vi "Read Occupied Queue.vi"(8 "error in (no error)":errorcluster, 11 "Circular Buffer 2D U16 DVR Queue Circular Buffer in":refnum<class "Circular Buffer 2D U16 DVR Queue Circular Buffer.lvclass">) -> (0 "error out":errorcluster, 2 "2D U16 DVR Queue":T1, 3 "Circular Buffer 2D U16 DVR Queue Circular Buffer out":refnum<class "Circular Buffer 2D U16 DVR Queue Circular Buffer.lvclass">)   [LabVIEW 2024, in "Circular Buffer 2D U16 DVR Queue Circular Buffer.lvclass"]
uses:
  Circular Buffer 2D U16 DVR Queue Circular Buffer.lvclass
  Type Def/2D U16 DVR Queue.ctl
  Type Def/2D U16 DVR.ctl
  Circular Buffer 2D U16 DVR Queue Circular Buffer.lvclass/Circular Buffer 2D U16 DVR Queue Circular Buffer.ctl
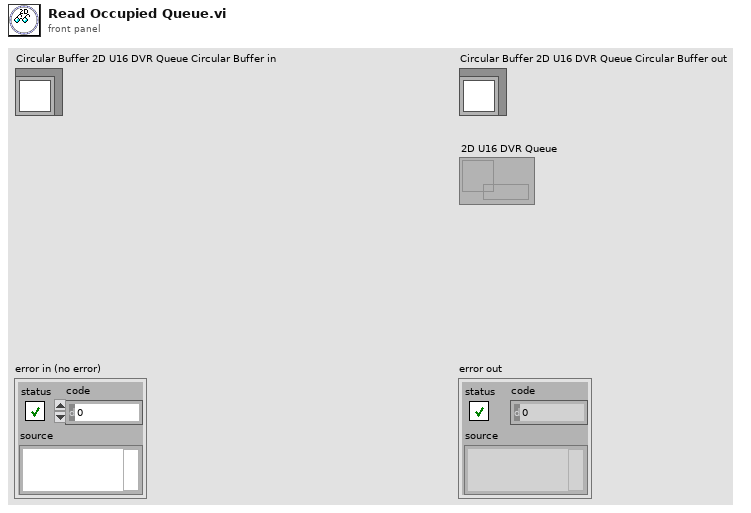
[diagram p1: front panel]
types:
  T1 = typedef "2D U16 DVR Queue.ctl" = refnum<queue>
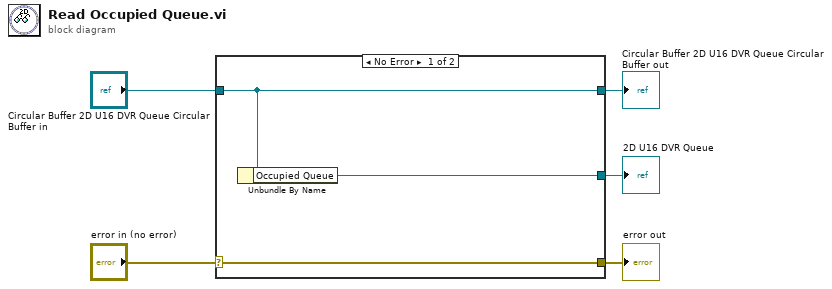
[diagram p0: block diagram]
diagram:
  n1 = case shown="No Error" "error in (no error)" {
    selector: "error in (no error)" -> [w8 w9]
    tunnel: [w8 w9] -> w4
    tunnel: [w7 w10] -> w2
    tunnel: "Circular Buffer 2D U16 DVR Queue Circular Buffer in" -> [w7 w10]
    tunnel: [w6 _] -> w1
    frame No Error {
      n2 = Unbundle By Name(w7) -> ("Occupied Queue"=w6:T1)
    }
    frame Error {
    }
  }
  "error out" <- w4
  "Circular Buffer 2D U16 DVR Queue Circular Buffer out" <- w2
  "2D U16 DVR Queue" <- w1
